vi "Графики-06-волны.vi"() -> ()   [LabVIEW 2017]
panel:
  out "Intensity Graph":dbl[][](graph)
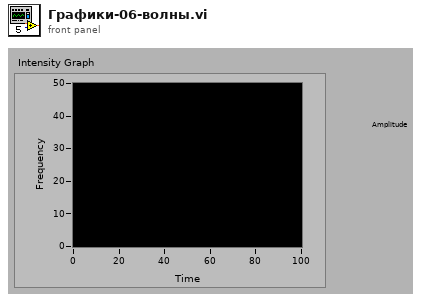
[diagram p1: front panel]
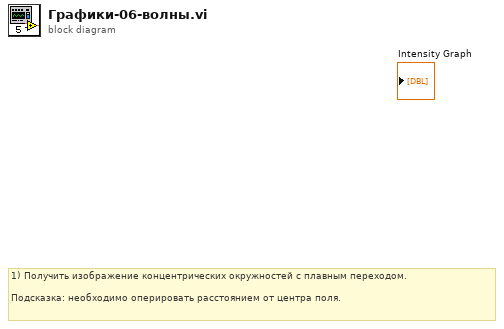
[diagram p0: block diagram]
diagram:
  # "1) Получить изображение концентрических окружностей с плавным переходом.\n\nПодсказка: необходимо оперировать расстоянием от центра поля."
